vi "Set Setpoint.vi"(8 "error in (no error)":errorcluster, 10 "Setpoint":i32, 11 "Eurotherm 3200 PID Controller in":refnum<class "Eurotherm 3200 PID Controller.lvclass">) -> (0 "error out":errorcluster, 3 "Eurotherm 3200 PID Controller out":refnum<class "Eurotherm 3200 PID Controller.lvclass">)   [LabVIEW 2011, in "Eurotherm 3200 PID Controller.lvclass"]
uses:
  Eurotherm 3200 PID Controller.lvclass
  Eurotherm 3200 PID Controller.lvclass/Eurotherm 3200 PID Controller.ctl
  <instrlib>/Eurotherm 32xx Series/Eurotherm 32xx Series.lvlib
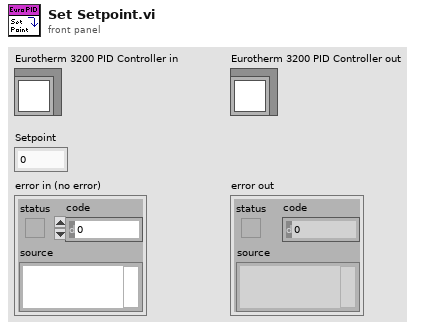
[diagram p1: front panel]
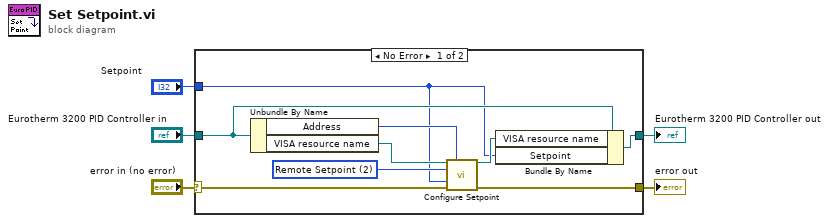
[diagram p0: block diagram]
diagram:
  n1 = case shown="No Error" "error in (no error)" {
    selector: "error in (no error)" -> [w11 w16]
    tunnel: [w10 w16] -> w4
    tunnel: [w7 w15] -> w2
    tunnel: "Eurotherm 3200 PID Controller in" -> [w9 w15]
    tunnel: "Setpoint" -> [w6 _]
    frame No Error {
      w13 = u8 2 items=["Setpoint 1", "Setpoint 2", "Remote Setpoint", "Target Setpoint"] ("Setpoint (0: Setpoint 1)")
      n2 = Unbundle By Name(w9) -> ("Address"=w12:u8, "VISA resource name"=w14:refnum<visa-resource-name>)
      n3 = call <instrlib>:"Configure Setpoint.vi"("VISA resource name"=w14, "Unit Address (1)"=w12, "Setpoint (0: Setpoint 1)"=w13, "Setpoint Value (0)"=w6, "error in (no error)"=w11) -> ("VISA resource name out"=w8:refnum<visa-resource-name>, "error out"=w10:errorcluster)  [unwired: 9 in]
      n4 = Bundle By Name(cluster=w9, "VISA resource name"=w8, "Setpoint"=w6) -> (w7:refnum<class "Eurotherm 3200 PID Controller.lvclass">)
    }
    frame Error {
    }
  }
  "error out" <- w4
  "Eurotherm 3200 PID Controller out" <- w2
